vi "oa_Check Params for Envelope Detection (Order).vi"(7 "reset":bool, 8 "error in (no error)":errorcluster, 9 "pulse/revolution (1)":i32=1, 10 "span [Order]":dbl, 11 "center":dbl) -> (0 "error out":errorcluster, 1 "pulse/revolution out":i32, 2 "span [Order] out":dbl, 3 "center out":dbl, 5 "reset out":bool)   [LabVIEW 2017, in "SoundVib_FaultAnalysis.lvlib"]
uses:
  <vilib>/addons/Sound and Vibration/Order Analysis/Fault Analysis/SoundVib_FaultAnalysis.lvlib
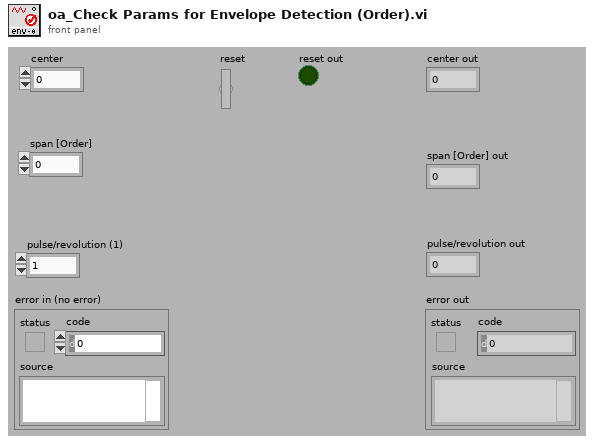
[diagram p1: front panel]
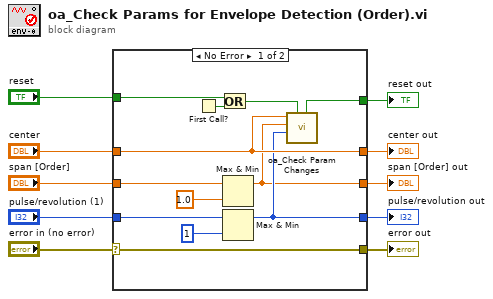
[diagram p0: block diagram]
diagram:
  n1 = case shown="No Error" "error in (no error)" {
    selector: "error in (no error)" -> [w22 w27]
    tunnel: [w22 w27] -> w9
    tunnel: "pulse/revolution (1)" -> [w16 w25]
    tunnel: "reset" -> [w19 w26]
    tunnel: [w17 w26] -> w7
    tunnel: [w12 w25] -> w6
    tunnel: "center" -> [w21 w24]
    tunnel: [w21 w24] -> w4
    tunnel: "span [Order]" -> [w13 w23]
    tunnel: [w11 w23] -> w1
    frame No Error {
      n2 = First Call?() -> (First Call?: T/F=w20:bool)
      n3 = Or(x=w19, y=w20) -> (x .or. y?=w18:bool)
      n4 = Max & Min(x=w13, y=1.0 ("x")) -> (max(x,y)=w11:dbl)  [unwired: 1 out]
      n5 = Max & Min(x=w16, y=1) -> (max(x,y)=w12:i32)  [unwired: 1 out]
      n6 = call <vilib>:"oa_Check Param Changes.vi"("Reset?"=w18, "param3"=w12, "param2"=w11, "param1"=w21) -> ("Reset out"=w17:bool)  [unwired: 7 in]
    }
    frame Error {
    }
  }
  "error out" <- w9
  "reset out" <- w7
  "pulse/revolution out" <- w6
  "center out" <- w4
  "span [Order] out" <- w1
